vi "Enable Limit Test Beeper.vi"(0 "VISA resource name":refnum<visa-resource-name>, 5 "Limit Test Number":u16=1 min=1 max=2 step=1, 7 "Function":u16(ring) items=["Voltage: DC", "Voltage: AC", "Current: DC", "Current: AC", "2W Resistance", "4W Resistance", "Diode", "Capacitance", "Temperature", "Continuity", "Frequency", "Period", "Ratio", "Digitize Voltage", "Digitize Current"], 9 "Beep When":u16(ring) items=["Never", "On Test Failure", "On Test Pass"], 11 "error in (no error)":errorcluster) -> (4 "VISA resource name out":refnum<visa-resource-name>, 15 "error out":errorcluster)   [LabVIEW 2021, in "Keithley DMM7510.lvlib"]
doc: "This VI enables or disables a beeper that sounds when a limit is exceeded."
uses:
  Keithley DMM7510.lvlib
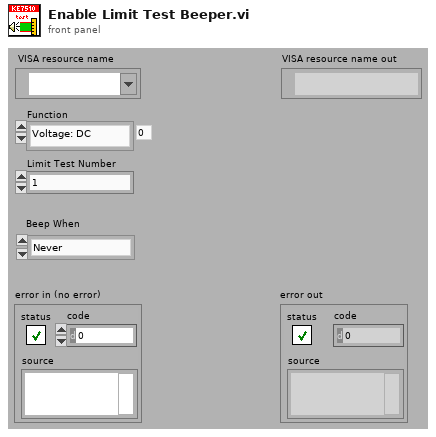
[diagram p1: front panel]
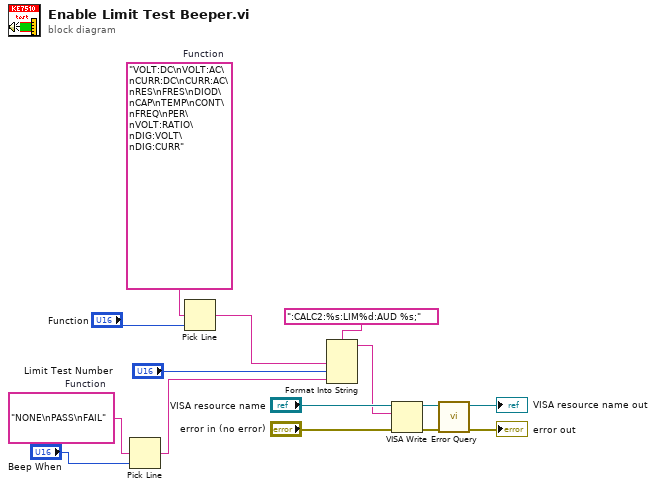
[diagram p0: block diagram]
diagram:
  w2 = "NONE\nPASS\nFAIL"  # Function
  w5 = "VOLT:DC\nVOLT:AC\nCURR:DC\nCURR:AC\nRES\nFRES\nDIOD\nCAP\nTEMP\nCONT\nFREQ\nPER\nVOLT:RATIO\nDIG:VOLT\nDIG:CURR"  # Function
  n1 = Pick Line(multi-line string=w2, line index="Beep When") -> (output string=w1:string)  [unwired: 1 out]
  n2 = Pick Line(multi-line string=w5, line index="Function") -> (output string=w7:string)  [unwired: 1 out]
  n3 = Format Into String(format string=":CALC2:%s:LIM%d:AUD %s;", w7, "Limit Test Number", w1) -> (resulting string=w8:string)  [unwired: 2 in, 1 out]
  n4 = VISA Write(VISA resource name="VISA resource name", write buffer=w8, error in (no error)="error in (no error)") -> (VISA resource name out=w11:refnum<visa-resource-name>, error out=w10:errorcluster)  [unwired: 1 out]
  n5 = call "Error Query.vi"("error in (no error)"=w10, "VISA resource name"=w11) -> ("error out"=→"error out":errorcluster, "VISA resource name out"=→"VISA resource name out":refnum<visa-resource-name>)  [unwired: 8 out]
